vi "写入固件.vi"(8 "错误输入":errorcluster, 10 "selected path":path, 11 "MB session in":refnum<class "MB_Master.lvclass">) -> (0 "error out":errorcluster, 2 "结果字符串":string, 3 "MB session out":refnum<class "MB_Master.lvclass">)   [LabVIEW 2016, in "斯坦道氟化物.lvlib"]
uses:
  <vilib>/Plasmionique/MB Master/MB_Master/MB_Master.lvclass
  <vilib>/NI/Progress Bar/Controls/Update Bar Actions.ctl
  <vilib>/Plasmionique/MB Master/MB_Master_Serial/MB_Master_Serial.lvclass
  C:/Program Files (x86)/National Instruments/LabVIEW 2016/vi.lib/Plasmionique/MB Master/MB_Master/MB_Master.lvclass
  <vilib>/Plasmionique/MB Master/MB Master.lvlib
  <vilib>/NI/Progress Bar/Progress Bar.lvlib
panel:
  out "数值":i32
  out "error out 2":errorcluster caption="error out"
  in  "引用选择":enum16{"MB引用", "自建引用"}(ring)
  in  "VISA Resource":refnum<visa-resource-name>
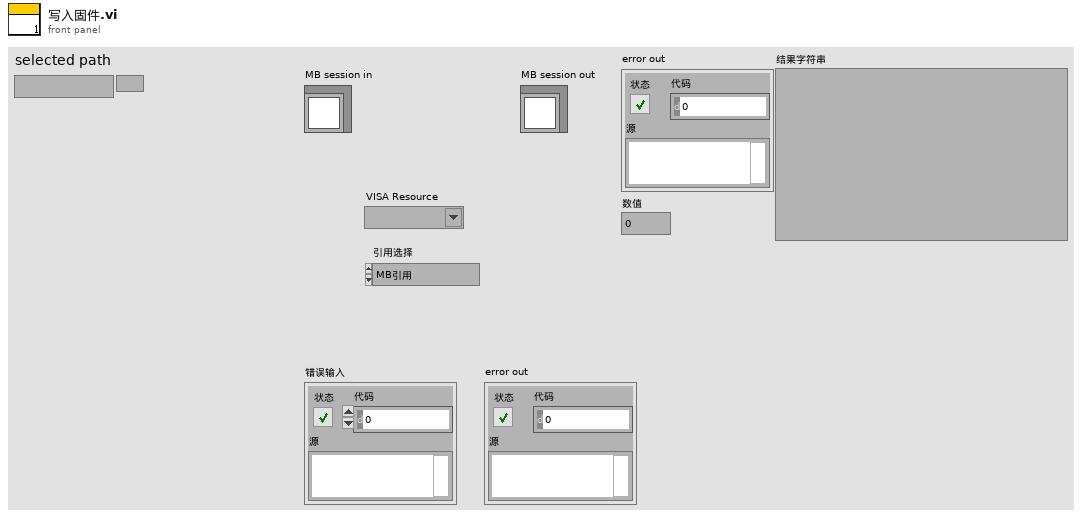
[diagram p1: front panel]
types:
  T1 = typedef "Progress Bar.lvlib/Update Bar Actions.ctl" = enum16{"Add To Existing", "Set to Value"}
  T2 = enum16{"open", "replace", "create", "open or create", "replace or create", "replace or create with confirmation"}
  T3 = enum16{"big-endian, network order", "native, host order", "little-endian"}
  T4 = cluster{"baud rate (bps)":u32, "stop bits":u16, "parity":u16, "flow control":u16, "timeout":u32, "retries":i32}
  T5 = typedef "SingleStepTestV3.lvlib/SingleStepTestV3.lvclass/仪器版本.ctl" = enum16{"A版", "B版", "A1版"}
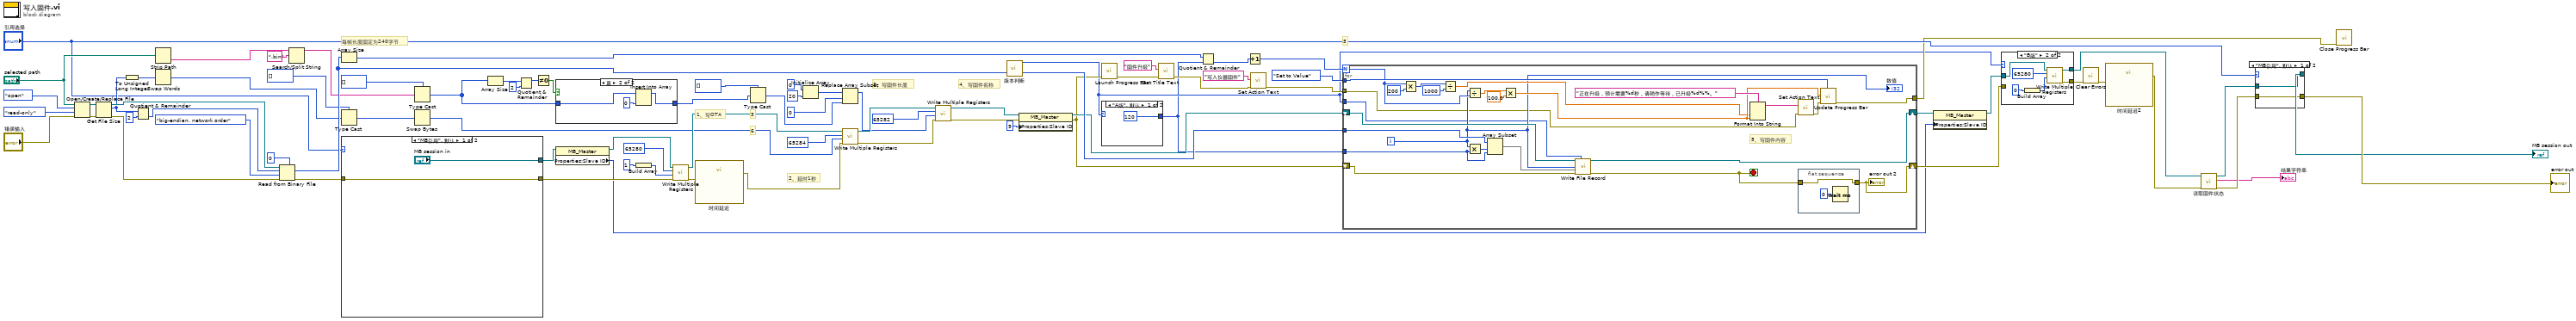
[diagram p0: block diagram]
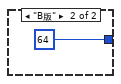
[diagram p2: hidden frame]
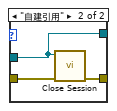
[diagram p5: hidden frame]
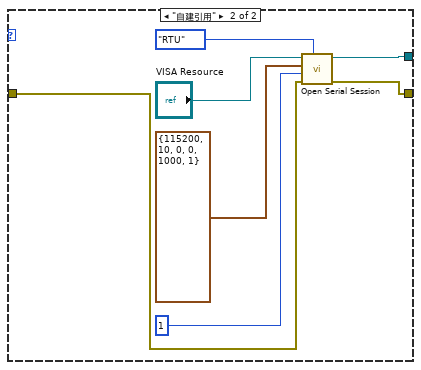
[diagram p6: hidden frame]
diagram:
  # "3"
  # "6"
  # "4、写固件名称"
  # "3、写固件长度"
  # "1、写OTA"
  # "5"
  # "每帧长度固定为240字节"
  # "2、延时1秒"
  n1 = Open/Create/Replace File(file path (use dialog)="selected path", error in="错误输入", operation (0:open)=T2."open" ("操作(0:open)"), access (0:read/write)=enum16{"read/write", "read-only", "write-only"}."read-only" ("权限(0:read/write)")) -> (refnum out=w72:refnum<file>, error out=w70:errorcluster)  [unwired: 2 in, 1 out]
  n2 = Get File Size(file=w72, error in=w70) -> (refnum out=w71:refnum<file>, size (in bytes)=w65:i64, 0:w69:errorcluster)
  n3 = To Unsigned Long Integer(number=w65) -> (unsigned 32bit integer=w46:u32)
  n4 = Quotient & Remainder(x=w65, y=i64 2) -> (floor(x/y)=w67:i64)  [unwired: 1 out]
  n5 = Strip Path(path="selected path") -> (name=w74:string)  [unwired: 1 out]
  n6 = Swap Words(1:w46) -> (0:w45:u32)
  n7 = Read from Binary File(5:u16 0, 8:w69, 9:T3."big-endian, network order" ("字节顺序(0:big-endian, network order)"), 10:w67, 11:w71) -> (0:w73:errorcluster, 2:w66:u16[])  [unwired: 1 in, 2 out]
  n8 = Search/Split String(string=w74, search string/char (-)=".bin" ("搜索字符串/字符(-)")) -> (substring before match=w55:string)  [unwired: 1 in, 2 out]
  n9 = Array Size(array=w66) -> (size(s)=w64:i32)
  n10 = Type Cast(type=u16[] [], x=w45) -> (*(type *) &x=w60:u16[])
  n11 = case shown="\"MB引用\", 默认" "引用选择" {
    tunnel: ["MB session in" w89] -> w11
    tunnel: w73 -> [w83 w88]
    tunnel: [w83 w87] -> w43
    frame "MB引用", Default {
    }
    frame "自建引用" {
      n12 = call <vilib>:"Open Serial Session.vi"("Mode (RTU)"=enum16{"RTU", "ASCII"}."RTU", "Error in"=w88, "Slave ID"=u8 1, "Serial Config"=T4 {"baud rate (bps)"=115200, "stop bits"=10, "parity"=0, "flow control"=0, "timeout"=1000, "retries"=1}, "VISA Resource"="VISA Resource") -> ("Error out"=w87:errorcluster, "MB_Serial session"=w89:refnum<class "MB_Master_Serial.lvclass">)  [unwired: 5 in]
    }
  }
  n13 = Type Cast(type=u8[] [], x=w55) -> (*(type *) &x=w38:u8[])
  n14 = Swap Bytes(anything=w60) -> (byte swapped=w36:u16[])
  n15 = Array Size(array=w38) -> (size(s)=w42:i32)
  n16 = Quotient & Remainder(x=w42, y=2) -> (x-y*floor(x/y)=w40:i32)  [unwired: 1 out]
  n17 = Not Equal To 0?(x=w40) -> (x != 0?=w39:bool)
  n18 = case shown="真" w39 {
    tunnel: w38 -> [w91 w94]
    tunnel: [w91 w93] -> w37
    frame False {
    }
    frame True {
      n19 = Insert Into Array(array=w94, new element=u8 0 ("新元素/子数组")) -> (w93:u8[])  [unwired: 1 in]
    }
  }
  n20 = property class="MB_Master"(reference=w11) -> (reference out=w10:refnum<class "MB_Master.lvclass">, "Properties:Slave ID"=w8:u8)  [unwired: 1 in, 1 out]
  n21 = Build Array(u16 1 ("value")) -> (w57:u16[])
  n22 = call <vilib>:"Write Multiple Registers.vi"("error in (no error)"=w43, "values"=w57, "starting address"=u16 65280, "MB session in"=w10) -> ("error out"=w62:errorcluster, "MB session out"=w52:refnum<class "MB_Master.lvclass">)  [unwired: 6 in]
  n23 = call "时间延迟"("error in (no error)"=w62) -> ("error out"=w53:errorcluster)  [unwired: 10 in]
  n24 = Type Cast(type=u16[] [], x=w37) -> (*(type *) &x=w17:u16[])
  n25 = Initialize Array(u16 0, 20 ("维数大小")) -> (w18:u16[])
  n26 = Replace Array Subset(array=w18, new element=w17, index=0 ("索引")) -> (w15:u16[])
  n27 = call <vilib>:"Write Multiple Registers.vi"("error in (no error)"=w53, "values"=w36, "starting address"=u16 65284, "MB session in"=w52) -> ("error out"=w23:errorcluster, "MB session out"=w24:refnum<class "MB_Master.lvclass">)  [unwired: 6 in]
  n28 = call <vilib>:"Write Multiple Registers.vi"("error in (no error)"=w23, "values"=w15, "starting address"=u16 65282, "MB session in"=w24) -> ("error out"=w47:errorcluster, "MB session out"=w50:refnum<class "MB_Master.lvclass">)  [unwired: 6 in]
  n29 = call "版本判断.vi"() -> ("仪器版本"=w7:T5)  [unwired: 11 in]
  n30 = property class="MB_Master"(reference=w50, error in=w47, "Properties:Slave ID"=u8 9 ("Slave ID")) -> (reference out=w48:refnum<class "MB_Master.lvclass">, error out=w26:errorcluster)
  n31 = call <vilib>:"Launch Progress Bar.vi"("error in (no error)"=w26) -> ("error out"=w29:errorcluster)  [unwired: 9 in, 1 out]
  n32 = case shown="\"A版\", 默认" w7 {
    tunnel: [120 ("y") 64 ("y")] -> w6
    frame "A版", Default {
    }
    frame "B版" {
    }
  }
  n33 = call <vilib>:"Set Title Text.vi"("error in (no error)"=w29, "Installer Title"="固件升级") -> ("error out"=w28:errorcluster)  [unwired: 9 in]
  n34 = Quotient & Remainder(x=w64, y=w6) -> (floor(x/y)=w35:i32)  [unwired: 1 out]
  n35 = Increment(x=w35) -> (x+1=w51:i32)
  n36 = call <vilib>:"Set Action Text.vi"("error in (no error)"=w28, "Action Text"="写入仪器固件") -> ("error out"=w31:errorcluster)  [unwired: 9 in]
  n37 = for {
    N: w51 -> [w105]
    shift-right: [w119] -> w14
    shift-left: w48 -> [w121]
    shift-right: [w101] -> w13
    shift-left: w26 -> [w120]
    tunnel: w66 -> [w117]
    tunnel: Update_Bar_Actions."Set to Value" ("Action") -> [w114]
    tunnel: [w113] -> w30
    tunnel: w31 -> [w99]
    tunnel: w7 -> [w98]
    tunnel: w6 -> [w97]
    i -> [w103]
    stop <- w102 stop-if-true
    # "5、写固件内容"
    n38 = Multiply(x=w105, y=200) -> (x*y=w109:i32)
    n39 = Divide(x=w109, y=u32 1000) -> (x/y=w106:dbl)
    n40 = Divide(x=w103, y=w105) -> (x/y=w110:dbl)
    n41 = Multiply(x=w103, y=w97) -> (x*y=w115:i32)
    n42 = Array Subset(array=w117, index=w115, length=w97) -> (w116:u16[])
    n43 = Multiply(x=w110, y=100.0) -> (x*y=w107:dbl)
    n44 = call "Write File Record.vi"("MB session in"=w121, "仪器版本"=w98, "Record Number"=w103, "values"=w116, "error in (no error)"=w120) -> ("MB session out"=w119:refnum<class "MB_Master.lvclass">, "error out"=w102:errorcluster)  [unwired: 9 in]
    n45 = Format Into String(format string="正在升级，预计需要%d秒，请稍作等待，已升级%d%%。" ("格式字符串"), w106, w107) -> (resulting string=w100:string)  [unwired: 2 in, 1 out]
    n46 = call <vilib>:"Set Action Text.vi"("error in (no error)"=w99, "Action Text"=w100) -> ("error out"=w112:errorcluster)  [unwired: 9 in]
    n47 = flat-sequence {
      tunnel: w102 -> [w123]
      tunnel: [w123] -> w101
      frame #0 {
        n48 = Wait (ms)(milliseconds to wait=u32 0 ("等待时间（毫秒）")) -> ()  [unwired: 1 out]
      }
    }
    n49 = call <vilib>:"Update Progress Bar.vi"("Action"=w114, "error in (no error)"=w112, "Value"=w107) -> ("error out"=w113:errorcluster)  [unwired: 8 in]
    "error out 2" <- w101
    "数值" <- w103
  }
  n50 = property class="MB_Master"(reference=w14, "Properties:Slave ID"=w8) -> (reference out=w9:refnum<class "MB_Master.lvclass">)  [unwired: 1 in, 1 out]
  n51 = case shown="\"B版\"" w7 {
    tunnel: w9 -> [w124 w128]
    tunnel: [w124 w127] -> w4
    tunnel: w13 -> [w125 _]
    tunnel: [w125 w126] -> w12
    frame "A版", Default {
    }
    frame "B版" {
      n52 = Build Array(0 ("value")) -> (w129:i32[])
      n53 = call <vilib>:"Write Multiple Registers.vi"("values"=w129, "starting address"=u16 65280, "MB session in"=w128) -> ("error out"=w126:errorcluster, "MB session out"=w127:refnum<class "MB_Master.lvclass">)  [unwired: 7 in]
    }
  }
  n54 = call <vilib>:"Clear Errors.vi"("error in (no error)"=w12) -> ("error out"=w34:errorcluster)  [unwired: 5 in, 1 out]
  n55 = call "时间延迟2"("error in (no error)"=w34) -> ("error out"=w5:errorcluster)  [unwired: 10 in]
  n56 = call "读取固件状态.vi"("错误输入"=w5, "MB session in"=w4) -> ("error out"=w2:errorcluster, "结果字符串"=→"结果字符串":string, "MB session out"=w3:refnum<class "MB_Master.lvclass">)  [unwired: 6 in, 1 out]
  n57 = case shown="\"MB引用\", 默认" "引用选择" {
    tunnel: w3 -> [w132 w134]
    tunnel: w2 -> [w133 w136]
    tunnel: [w133 w135] -> w80
    tunnel: [w132 w134] -> w33
    frame "MB引用", Default {
    }
    frame "自建引用" {
      n58 = call-dynamic "Close Session.vi"("error in (no error)"=w136, "MB session in"=w134) -> ("error out"=w135:errorcluster)  [unwired: 9 in]
    }
  }
  "error out" <- w80
  "MB session out" <- w33
  n59 = call <vilib>:"Close Progress Bar.vi"("error in (no error)"=w30) -> ()  [unwired: 9 in, 2 out]
